vi "FPGAcode4_Test1.vi"() -> ()   [LabVIEW 2015]
uses:
  Limits_In.ctl
  Discard_Points.ctl
  Filter_Cluster.ctl
  <vilib>/Platform/TimedLoop/XDataNode/timing_clust.ctl
  <vilib>/Platform/TimedLoop/XDataNode/nitl_modes.ctl
  <vilib>/Platform/TimedLoop/XDataNode/wakeup.ctl
  Detector_Cluster.ctl
  Correlations.ctl
  <vilib>/rvi/Emulation/niFpgaGetClockAttributes.vi
  <vilib>/rvi/Emulation/niFpgaSctlEmulationGetInTimedLoop.vi
  <vilib>/rvi/Emulation/niFpgaEmulationReportErrorSimple.vi
  <vilib>/rvi/Emulation/niFpgaProcessEmulError.vi
  <vilib>/rvi/eio/common/nirviEmuTemplateMethod_errors.vi
  <vilib>/rvi/Emulation/niFpgaCriticalErrorInLSC.vi
  <vilib>/eio/EIONode/EIONode.xnode
  <vilib>/Platform/TimedLoop/XDataNode/XDataNode.xnode
  <vilib>/Platform/TimedLoop/XDataNode/XDNodeRunTimeDep.lvlib
panel:
  out "Charge":T1
  out "Mass":T2
  out "Velocity Count":T3
  in  "User Trigger Distance":fxp<+/-,34,18>
  out "User Trigger":bool
  out "Particles Discarded":i16
  out "All Discard Points":T4
  in  "Boxcar 3 Size Factor":fxp<+/-,32,16>=0.1999969482421875 format="%.2g"
  in  "Charge Error Factor":fxp<+/-,32,16>=1.100006103515625 format="%.2g"
  in  "Max Correlation Factor":fxp<+,32,4>=0.25 format="%.3g"
  in  "Threshold Factor":fxp<+/-,32,16>=1.0 format="%.2g"
  out "DCS 2":bool
  out "Detectors":cluster{"Det 1":i16, "Det 3":i16}
  out "DCS 1":bool
  in  "Limits":T6
  in  "Calibrate":bool=TRUE
  in  "Armed":bool
  out "Plates":bool
  in  "One Shot":bool
  # "These factors above are in the front\npanel so it is possible to experiment\nwith many different configurations\nof the FPGA on the fly. One can even\nchange the relative size of one filter."
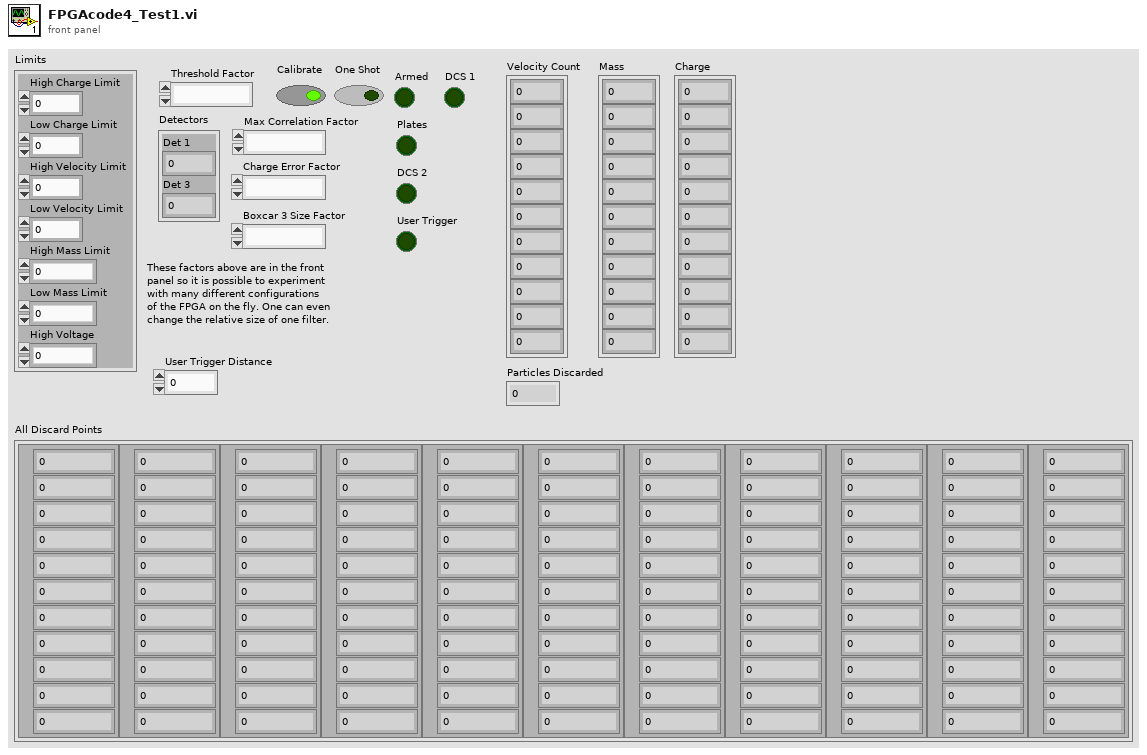
[diagram p1: front panel]
types:
  T1 = cluster{"[0]":fxp<+/-,64,-10>, "[1]":fxp<+/-,64,-10>, "[2]":fxp<+/-,64,-10>, "[3]":fxp<+/-,64,-10>, "[4]":fxp<+/-,64,-10>, "[5]":fxp<+/-,64,-10>, "[6]":fxp<+/-,64,-10>, "[7]":fxp<+/-,64,-10>, "[8]":fxp<+/-,64,-10>, "[9]":fxp<+/-,64,-10>, "[10]":fxp<+/-,64,-10>}
  T2 = cluster{"[0]":fxp<+/-,64,-2>, "[1]":fxp<+/-,64,-2>, "[2]":fxp<+/-,64,-2>, "[3]":fxp<+/-,64,-2>, "[4]":fxp<+/-,64,-2>, "[5]":fxp<+/-,64,-2>, "[6]":fxp<+/-,64,-2>, "[7]":fxp<+/-,64,-2>, "[8]":fxp<+/-,64,-2>, "[9]":fxp<+/-,64,-2>, "[10]":fxp<+/-,64,-2>}
  T3 = cluster{"[0]":i32, "[1]":i32, "[2]":i32, "[3]":i32, "[4]":i32, "[5]":i32, "[6]":i32, "[7]":i32, "[8]":i32, "[9]":i32, "[10]":i32}
  T4 = typedef "Discard_Points.ctl" = cluster{"Discard Points 1":T5, "Discard Points 2":T5, "Discard Points 3":T5, "Discard Points 4":T5, "Discard Points 5":T5, "Discard Points 6":T5, "Discard Points 7":T5, "Discard Points 8":T5, "Discard Points 9":T5, "Discard Points 10":T5, "Discard Points 11":T5}
  T5 = typedef "Filter_Cluster.ctl" = cluster{"1":i32, "2":i32, "3":i32, "4":i32, "5":i32, "6":i32, "7":i32, "8":i32, "9":i32, "10":i32, "11":i32}
  T6 = typedef "Limits_In.ctl" = cluster{"High Charge Limit":fxp<+,32,-41>, "Low Charge Limit":fxp<+,32,-41>, "High Velocity Limit":fxp<+,18,18>, "Low Velocity Limit":fxp<+,18,18>, "High Mass Limit":fxp<+/-,33,-35>, "Low Mass Limit":fxp<+/-,33,-35>, "High Voltage":fxp<+,16,22>}
  T7 = typedef "Detector_Cluster.ctl" = cluster{"Det 1":i32, "Det 2":i32}
  T8 = cluster{"Filter 1":T7, "Filter 2":T7, "Filter 3":T7, "Filter 4":T7}
  T9 = cluster{"Distance to PSU":fxp<+/-,32,5>, "Distance to end of PSU":fxp<+/-,32,5>, "Distance to DCS 2":fxp<+/-,32,5>, "Distance to DCS 1":fxp<+/-,32,5>, "Distance to front of LEIL Chamber":fxp<+/-,32,5>}
  T10 = cluster{"Detector Max Speed Count":i32, "Detector Min Speed Count":i32, "Gap Max Speed Count":i32, "Gap Min Speed Count":i32}
  T11 = cluster{"Distance to PSU":fxp<+/-,64,22>, "Distance to end of PSU":fxp<+/-,64,22>, "Distance to DCS 2":fxp<+/-,64,22>, "Distance to DCS 1":fxp<+/-,64,22>, "Distance to front of LEIL Chamber":fxp<+/-,64,22>}
  T12 = typedef "XDNodeRunTimeDep.lvlib/timing_clust.ctl" = cluster{"Expected End [f-1]":u64, "Actual End [f-1]":u64, "Finished Late? [f-1]":bool, "Expected End [i-1]":u64, "Actual End [i-1]":u64, "Finished Late? [i-1]":bool, "Expected Start [i]":u64, "Actual Start [i]":u64, "Expected Start [f]":u64, "Actual Start [f]":u64, "Source Name":string, "Structure Name":string, "Period":i64, "Deadline":i64, "Offset":i64, "Start":i64, "Priority":i32, "Timeout":i32, "Mode":T13, "Wakeup Reason":T14, "Error":errorcluster, "Source Type":string, "Secondary Source Type":string, "Global End Time":u64, "Global Start Time":u64, "Frame Duration":u64, "Iteration Duration":u64, "Assigned CPU":i32, "I/O Scan Engine Mode":u32}
  T13 = typedef "XDNodeRunTimeDep.lvlib/nitl_modes.ctl" = enum32{"No Change", "Process missed periods, maintain original phase", "Discard missed periods, maintain original phase", "Process missed periods, ignore original phase", "Discard missed periods, ignore original phase"}
  T14 = typedef "XDNodeRunTimeDep.lvlib/wakeup.ctl" = enum32{"Normal", "Aborted", "Asynchronous wakeup", "Timing source error", "Timed loop error", "Timeout"}
  T15 = cluster{"Filter 1":T7, "Filter 2":T7, "Filter 3":T7, "Filter 4":T7}[]
  T16 = cluster{"Distance to PSU":i32, "Distance to end of PSU":i32, "Distance to DCS 2":i32, "Distance to DCS 1":i32, "Distance to front of LEIL Chamber":i32}
  T17 = typedef "Correlations.ctl" = cluster{"First Correlation":i32, "Latest Correlation":i32}
  T18 = cluster{"First Detector Count":i32, "Detector Gap Count":i32, "Second Detector Count":i32, "Second Detector Final Count":i32}
  T19 = cluster{"Detectors":cluster{"Det 1":i16, "Det 3":i16}, cluster{"Det 1":i16, "Det 2":i16}, cluster{"Det 1":i16, "Det 2":i16}, cluster{"Det 1":i16, "Det 2":i16}}
  T20 = cluster{cluster{"Det 1":i16, "Det 2":i16}, cluster{"Det 1":i16, "Det 2":i16}, cluster{"Det 1":i16, "Det 2":i16}, cluster{"Det 1":i16, "Det 2":i16}}
  T21 = cluster{"[0]":u8, "[1]":u8, "[2]":u8, "[3]":u8, "[4]":u8, "[5]":u8, "[6]":u8, "[7]":u8, "[8]":u8, "[9]":u8, "[10]":u8}
  T22 = cluster{"All Discard Points[0]":T5, "All Discard Points[1]":T5, "All Discard Points[2]":T5, "All Discard Points[3]":T5, "All Discard Points[4]":T5, "All Discard Points[5]":T5, "All Discard Points[6]":T5, "All Discard Points[7]":T5, "All Discard Points[8]":T5, "All Discard Points[9]":T5, "All Discard Points[10]":T5}
  T23 = cluster{i32[], fxp<+/-,64,-2>[], fxp<+/-,64,-10>[]}
  T24 = cluster{"IO Module\\AI 0":i16, "IO Module\\AI 1":i16}
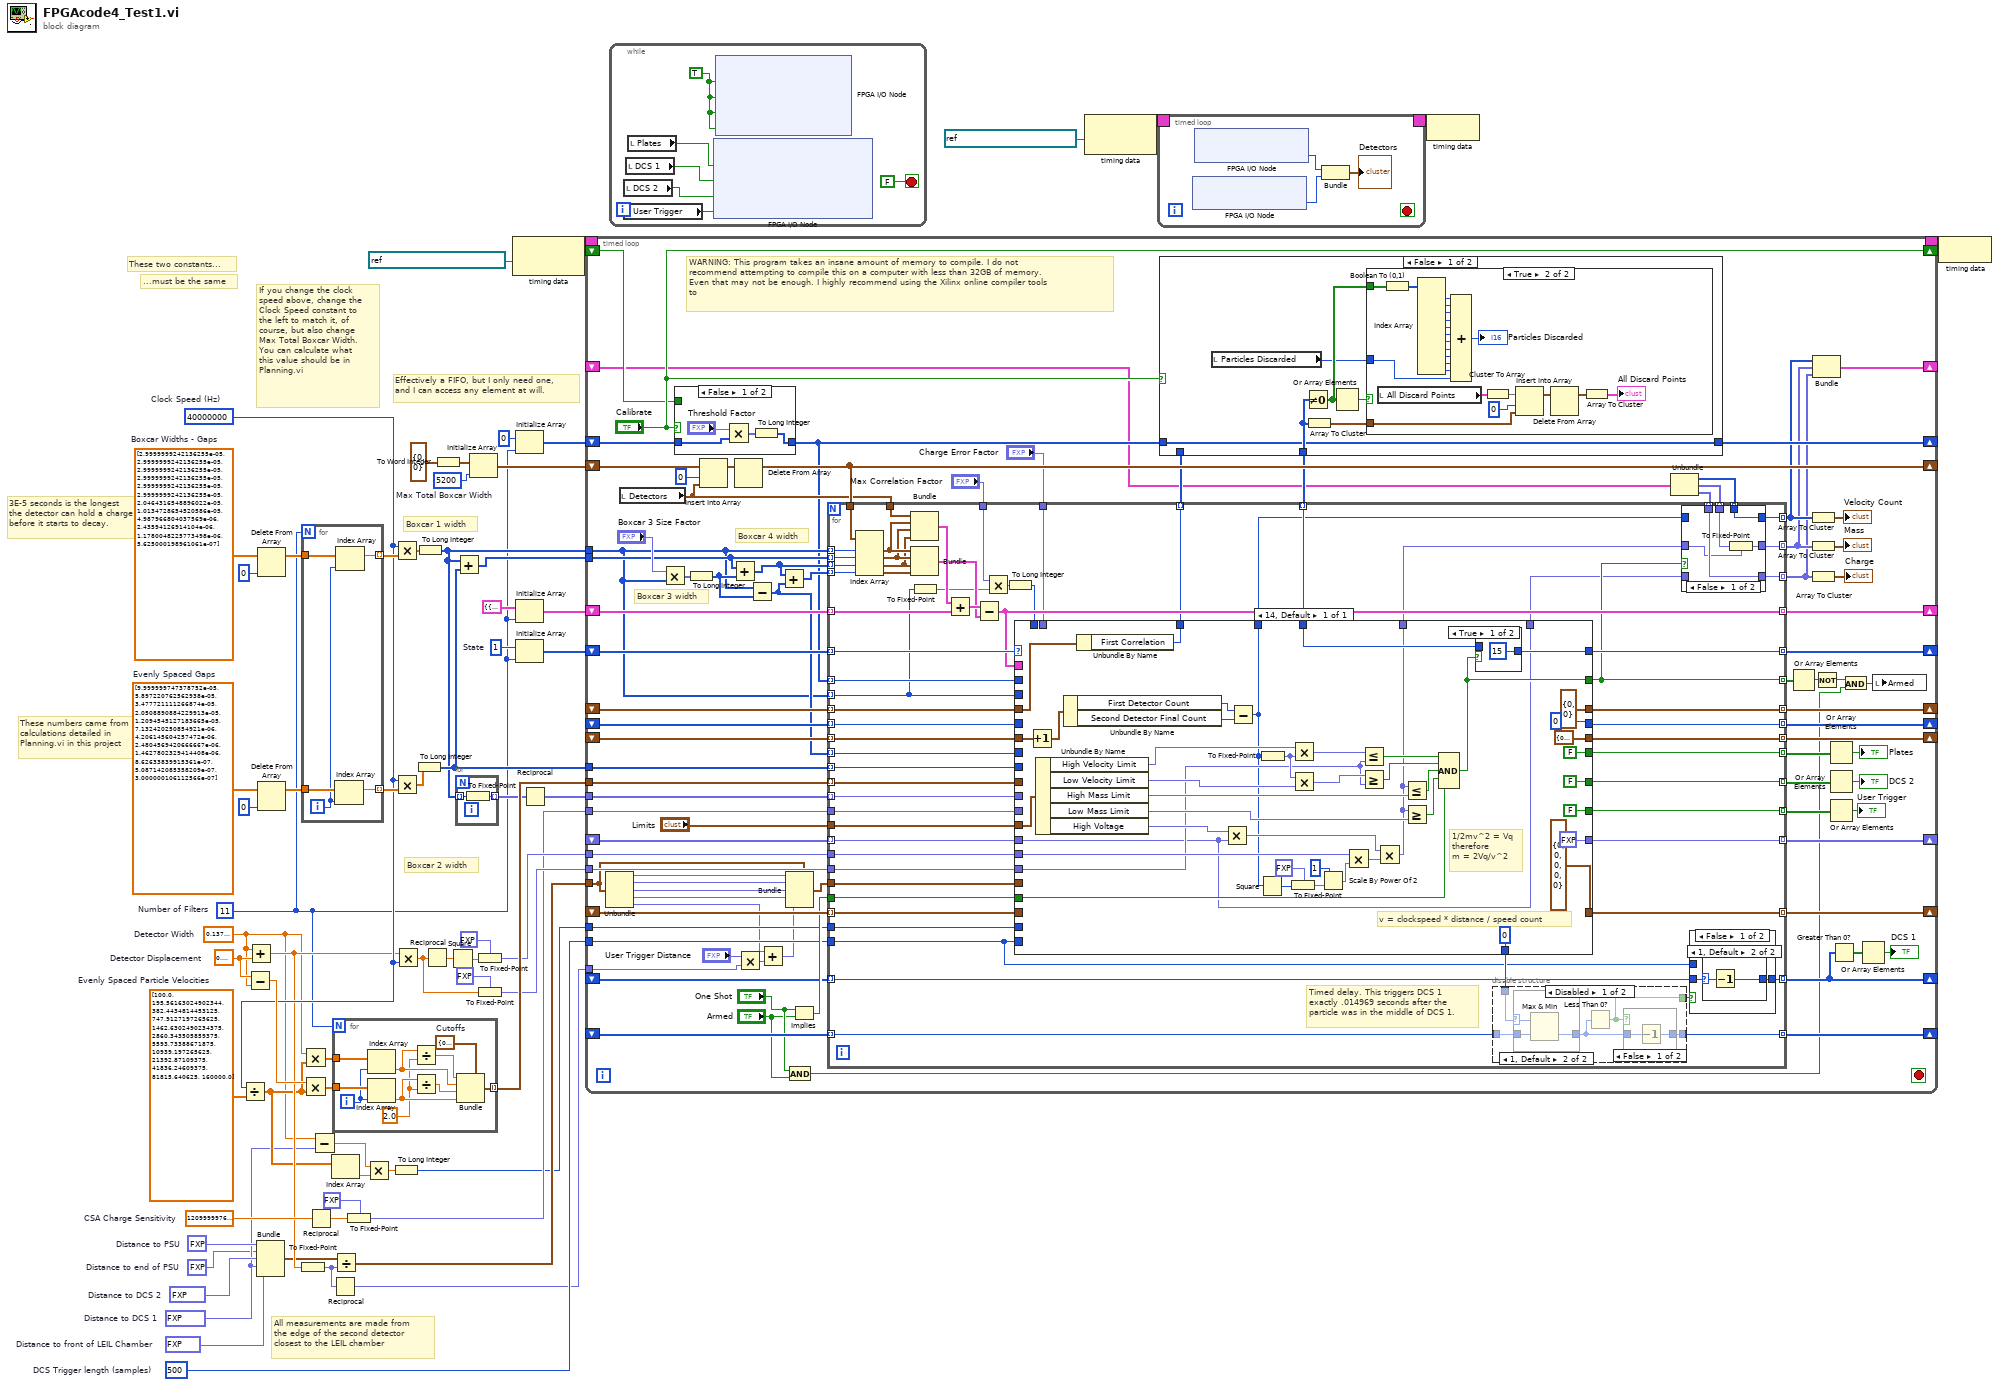
[diagram p0: block diagram]
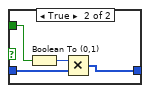
[diagram p2: hidden frame]
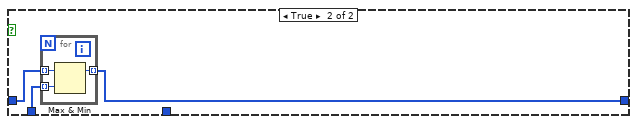
[diagram p4: hidden frame]
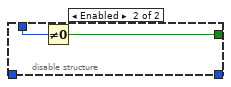
[diagram p10: hidden frame]
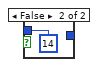
[diagram p11: hidden frame]
diagram:
  w1 = fxp<+/-,32,5> 4.297679997980595  # Distance to front of LEIL Chamber
  w7 = u16 500  # DCS Trigger length (samples)
  w12 = fxp<+/-,32,5> -1.3589000031352043  # Distance to DCS 1
  w16 = fxp<+/-,32,5> 2.6162000000476837  # Distance to DCS 2
  w4 = fxp<+/-,32,5> 1.8999999985098839  # Distance to end of PSU
  w17 = fxp<+/-,32,5> 1.5  # Distance to PSU
  w30 = sgl 12100000000000.0  # CSA Charge Sensitivity
  w52 = u8 1  # State
  w13 = sgl 0.6  # Detector Displacement
  w58 = sgl[] [3e-05, 3e-05, 3e-05, 3e-05, 3e-05, 3e-05, 2.0464317e-05, 1.0134729e-05, 4.987967e-06, 2.4359413e-06, 1.1780048e-06, 5.625e-07]  # Boxcar Widths - Gaps
  w56 = sgl[] [0.0001, 5.8972208e-05, 3.477721e-05, 2.050889e-05, 1.2094545e-05, 7.1324203e-06, 4.2061456e-06, 2.480457e-06, 1.4627802e-06, 8.6263384e-07, 5.087142e-07, 3e-07]  # Evenly Spaced Gaps
  w36 = sgl[] [100.0, 195.56163, 382.44348, 747.9127, 1462.6302, 2860.3435, 5593.734, 10939.197, 21392.871, 41836.246, 81815.64, 160000.0]  # Evenly Spaced Particle Velocities
  w33 = 40000000  # Clock Speed (Hz)
  w8 = sgl 0.138  # Detector Width
  w60 = 5200  # Max Total Boxcar Width
  w5 = 11  # Number of Filters
  # "...must be the same"
  # "These two constants..."
  # "If you change the clock\nspeed above, change the\nClock Speed constant to\nthe left to match it, of\ncourse, but also change\nMax Total Boxcar Width.\nYou can calculate what\nthis value should be in\nPlanning.vi"
  # "All measurements are made from\nthe edge of the second detector\nclosest to the LEIL chamber"
  # "Effectively a FIFO, but I only need one,\nand I can access any element at will."
  # "Boxcar 2 width"
  # "Boxcar 1 width"
  # "3E-5 seconds is the longest\nthe detector can hold a charge\nbefore it starts to decay."
  # "These numbers came from\ncalculations detailed in\nPlanning.vi in this project"
  n1 = Divide(x=w33, y=w36) -> (x/y=w14:sgl[])
  n2 = Subtract(x=w13, y=w8) -> (x-y=w35:sgl)
  n3 = Add(x=w8, y=w13) -> (x+y=w22:sgl)
  n4 = Bundle("Distance to PSU"=w17, "Distance to end of PSU"=w4, "Distance to DCS 2"=w16, "Distance to DCS 1"=w12, "Distance to front of LEIL Chamber"=w1) -> (w21:T9)  [unwired: 1 in]
  n5 = Delete From Array(array=w58, index=0) -> (array with subset deleted=w45:sgl[])  [unwired: 1 in, 1 out]
  n6 = Delete From Array(array=w56, index=0) -> (array with subset deleted=w47:sgl[])  [unwired: 1 in, 1 out]
  n7 = To Fixed-Point(number=w22) -> (fixed-point=w3:fxp<+/-,32,16>)  [unwired: 1 in]
  n8 = for {
    N: w5 -> [_]
    tunnel: w47 -> [w72]
    tunnel: [w69] -> w46 mode=indexing
    tunnel: w45 -> [w71]
    tunnel: [w70] -> w44 mode=indexing
    i -> [w68]
    n9 = Index Array(array=w72, index=w68) -> (element=w69:sgl)
    n10 = Index Array(array=w71, index=w68) -> (element=w70:sgl)
  }
  n11 = Multiply(x=w8, y=w14) -> (x*y=w54:sgl[])
  n12 = Multiply(x=w35, y=w14) -> (x*y=w55:sgl[])
  n13 = Reciprocal(x=w30) -> (1/x=w24:sgl)
  n14 = Subtract(x=w8, y=w12) -> (x-y=w10:sgl)
  n15 = Index Array(array=w14) -> (element=w11:sgl)  [unwired: 1 in]
  n16 = Reciprocal(x=w3) -> (1/x=w2:fxp<+/-,34,18>)
  n17 = for {
    N: w5 -> [_]
    tunnel: w55 -> [w82]
    tunnel: w54 -> [w81]
    tunnel: [w80] -> w49 mode=indexing
    i -> [w79]
    w73 = sgl 2.0 ("y")
    w78 = T10 {"Detector Max Speed Count"=0, "Detector Min Speed Count"=0, "Gap Max Speed Count"=0, "Gap Min Speed Count"=0}  # Cutoffs
    n18 = Index Array(array=w81, index=w79) -> (element=w77:sgl)
    n19 = Index Array(array=w82, index=w79) -> (element=w74:sgl)
    n20 = Divide(x=w77, y=w73) -> (x/y=w76:sgl)
    n21 = Divide(x=w74, y=w73) -> (x/y=w75:sgl)
    n22 = Bundle(cluster=w78, "Detector Max Speed Count"=w76, "Detector Min Speed Count"=w77, "Gap Max Speed Count"=w75, "Gap Min Speed Count"=w74) -> (w80:T10)
  }
  n23 = Divide(x=w21, y=w3) -> (x/y=w20:T11)
  n24 = To Fixed-Point(fixed-point type=fxp<+,32,-43> 0.0, number=w24) -> (fixed-point=w23:fxp<+,32,-43>)
  n25 = Multiply(x=w10, y=w11) -> (x*y=w9:sgl)
  n26 = To Long Integer(number=w9) -> (32bit integer=w6:i32)
  n27 = Multiply(x=w33, y=w44) -> (x*y=w48:sgl[])
  n28 = Multiply(x=w33, y=w46) -> (x*y=w53:sgl[])
  n29 = Multiply(x=w22, y=w33) -> (x*y=w27:sgl)
  n30 = To Long Integer(number=w53) -> (32bit integer=w43:i32[])
  n31 = To Long Integer(number=w48) -> (32bit integer=w39:i32[])
  n32 = Reciprocal(x=w27) -> (1/x=w32:sgl)
  n33 = To Word Integer(number=T7 {"Det 1"=0, "Det 2"=0} ("Detectors")) -> (16bit integer=w42:cluster{"Det 1":i16, "Det 2":i16})
  n34 = Square(x=w32) -> (x^2=w31:sgl)
  n35 = Add(x=w39, y=w43) -> (x+y=w15:i32[])
  n36 = for {
    tunnel: w39 -> [w84] mode=indexing
    tunnel: [w83] -> w38 mode=indexing
    n37 = To Fixed-Point(number=w84) -> (fixed-point=w83:fxp<+/-,32,32>)  [unwired: 1 in]
  }
  n38 = Initialize Array(w42, w60) -> (w61:cluster{"Det 1":i16, "Det 2":i16}[])
  n39 = To Fixed-Point(fixed-point type=fxp<+/-,32,-45> 0.0, number=w31) -> (fixed-point=w34:fxp<+/-,32,-45>)
  n40 = To Fixed-Point(fixed-point type=fxp<+,32,32> 0.0, number=w27) -> (fixed-point=w25:fxp<+,32,32>)
  n41 = node-c288(refnum<k21> "40 MHz Onboard Clock" ("Source Name")) -> (w64:T12)
  n42 = Initialize Array(0 ("element"), w5) -> (w18:i32[])
  n43 = Initialize Array(T8 {"Filter 1"={"Det 1"=0, "Det 2"=0}, "Filter 2"={"Det 1"=0, "Det 2"=0}, "Filter 3"={"Det 1"=0, "Det 2"=0}, "Filter 4"={"Det 1"=0, "Det 2"=0}} ("cluster"), w5) -> (w50:T15)
  n44 = Initialize Array(w52, w5) -> (w51:u8[])
  n45 = Reciprocal(x=w38) -> (1/x=w37:fxp<+/-,34,2>[])
  n46 = timed-loop {
    timing: w64 -> [_]
    timing-out: [_] -> w63
    shift-right: [w168] -> _
    shift-left: w61 -> [w171]
    shift-right: [w167] -> _
    shift-left: w50 -> [w160]
    shift-right: [w165] -> _
    shift-left: w51 -> [w166]
    shift-right: [w164] -> _
    shift-left: _ -> [w163]
    shift-right: [w162] -> _
    shift-left: _ -> [w161]
    tunnel: w49 -> [w158]
    shift-right: [w157] -> _
    shift-left: _ -> [w156]
    tunnel: w39 -> [w145]
    tunnel: w15 -> [w151]
    tunnel: w43 -> [w146]
    tunnel: w37 -> [w144]
    shift-right: [w142] -> _
    shift-left: _ -> [w141]
    tunnel: w34 -> [w140]
    tunnel: w23 -> [w139]
    tunnel: w25 -> [w138]
    tunnel: w20 -> [w116]
    shift-right: [w137] -> _
    shift-left: _ -> [w136]
    shift-right: [w134] -> _
    shift-left: w18 -> [w132]
    shift-right: ["Calibrate"] -> _
    shift-left: _ -> [w129]
    tunnel: w7 -> [w127]
    tunnel: w6 -> [w126]
    shift-right: [w123] -> _
    shift-left: _ -> [w125]
    shift-right: [w121] -> _
    shift-left: _ -> [w120]
    tunnel: w2 -> [w119]
    shift-right: [w90] -> _
    shift-left: _ -> [w89]
    stop <- _ stop-if-true
    # "WARNING: This program takes an insane amount of memory to compile. I do not\nrecommend attempting to compile this on a computer with less than 32GB of memory.\nEven that may not be enough. I highly recommend using the Xilinx online compiler tools\nto"
    # "Boxcar 3 width"
    # "Boxcar 4 width"
    n47 = Unbundle(w116) -> ("Distance to PSU"=w117:fxp<+/-,64,22>, "Distance to end of PSU"=w115:fxp<+/-,64,22>, "Distance to DCS 2"=w114:fxp<+/-,64,22>, "Distance to DCS 1"=w111:fxp<+/-,64,22>, "Distance to front of LEIL Chamber"=w110:fxp<+/-,64,22>)
    n48 = local read "Detectors"() -> (w159:cluster{"Det 1":i16, "Det 3":i16})
    n49 = Multiply(x="Boxcar 3 Size Factor", y=w145) -> (x*y=w153:fxp<+/-,64,48>[])
    n50 = case shown="False" "Calibrate" {
      tunnel: w132 -> [w173 w179]
      tunnel: [w172 w177] -> w131
      tunnel: w129 -> [_ w178]
      frame False {
        n51 = Multiply(x="Threshold Factor", y=w173) -> (x*y=w174:fxp<+/-,64,48>[])
        n52 = To Long Integer(number=w174) -> (32bit integer=w172:i32[])
      }
      frame True {
        n53 = Boolean To (0,1)(Boolean=w178) -> (0, 1=w176:i16)
        n54 = Multiply(x=w176, y=w179) -> (x*y=w177:i32[])
      }
    }
    n55 = To Long Integer(number=w153) -> (32bit integer=w154:i32[])
    n56 = Insert Into Array(array=w171, index=0, new element=w159) -> (w170:cluster{"Det 1":i16, "Det 2":i16}[])
    n57 = Add(x=w151, y=w154) -> (x+y=w150:i32[])
    n58 = Delete From Array(array=w170) -> (array with subset deleted=w168:cluster{"Det 1":i16, "Det 2":i16}[])  [unwired: 2 in, 1 out]
    n59 = Multiply(x="User Trigger Distance", y=w119) -> (x*y=w112:fxp<+/-,64,34>)
    n60 = Subtract(x=w145, y=w154) -> (x-y=w148:i32[])
    n61 = Add(x=w110, y=w112) -> (x+y=w109:fxp<+/-,64,35>)
    n62 = Add(x=w150, y=w148) -> (x+y=w149:i32[])
    n63 = Bundle(cluster=w116, "Distance to PSU"=w117, "Distance to end of PSU"=w115, "Distance to DCS 2"=w114, "Distance to DCS 1"=w111, "Distance to front of LEIL Chamber"=w109) -> (w113:T11)
    n64 = And(x="One Shot", y="Armed") -> (x .and. y?=w99:bool)
    n65 = Implies(1:"Armed", 2:"One Shot") -> (0:w128:bool)
    n66 = Unbundle(w89) -> (w88:i32[], w87:fxp<+/-,64,-2>[], w86:fxp<+/-,64,-10>[])
    n67 = for {
      tunnel: w168 -> [w280]
      tunnel: [w263] -> w167 mode=indexing
      tunnel: w166 -> [w279] mode=indexing
      tunnel: [w277] -> w165 mode=indexing
      tunnel: w131 -> [w278] mode=indexing
      tunnel: [w276] -> w164 mode=indexing
      tunnel: w163 -> [w275] mode=indexing
      tunnel: [w274] -> w162 mode=indexing
      tunnel: w161 -> [w273] mode=indexing
      tunnel: w160 -> [w267] mode=indexing
      tunnel: w159 -> [w272]
      tunnel: w158 -> [w262] mode=indexing
      tunnel: [w261] -> w157 mode=indexing
      tunnel: w156 -> [w260] mode=indexing
      tunnel: w145 -> [w259] mode=indexing
      tunnel: w151 -> [w258] mode=indexing
      tunnel: w150 -> [w257] mode=indexing
      tunnel: w149 -> [w256] mode=indexing
      tunnel: w145 -> [w216] mode=indexing
      tunnel: "Max Correlation Factor" -> [w255]
      tunnel: w148 -> [w254] mode=indexing
      tunnel: w146 -> [w253] mode=indexing
      tunnel: "Charge Error Factor" -> [w252]
      tunnel: [w251] -> w135 mode=indexing
      tunnel: w144 -> [w250] mode=indexing
      tunnel: "Limits" -> [w249]
      tunnel: [w248] -> w142 mode=indexing
      tunnel: w141 -> [w247] mode=indexing
      tunnel: w140 -> [w246]
      tunnel: w139 -> [w245]
      tunnel: w138 -> [w244]
      tunnel: w113 -> [w243]
      tunnel: [w242] -> w137 mode=indexing
      tunnel: w136 -> [w241] mode=indexing
      tunnel: [w240] -> w133 mode=indexing
      tunnel: w128 -> [w239]
      tunnel: w127 -> [w236]
      tunnel: w126 -> [w238]
      tunnel: [w235] -> w123 mode=indexing
      tunnel: w125 -> [w234] mode=indexing
      tunnel: [w232] -> w121 mode=indexing
      tunnel: w120 -> [w231] mode=indexing
      tunnel: [w230] -> w108 mode=indexing
      tunnel: [w229] -> w106 mode=indexing
      tunnel: [w228] -> w105 mode=indexing
      tunnel: [w227] -> w102 mode=indexing
      tunnel: [w221] -> w93 mode=indexing
      tunnel: [w226] -> w91 mode=indexing
      tunnel: [w224] -> w92 mode=indexing
      tunnel: w88 -> [w220] mode=indexing
      tunnel: w87 -> [w219] mode=indexing
      tunnel: w86 -> [w218] mode=indexing
      # "Timed delay. This triggers DCS 1\nexactly .014969 seconds after the\nparticle was in the middle of DCS 1."
      n68 = Index Array(array=w280, index #1=w259, index #2=w258, index #3=w257, index #4=w256) -> (element #1=w270:cluster{"Det 1":i16, "Det 2":i16}, element #2=w269:cluster{"Det 1":i16, "Det 2":i16}, element #3=w268:cluster{"Det 1":i16, "Det 2":i16}, element #4=w271:cluster{"Det 1":i16, "Det 2":i16})
      n69 = Bundle("Detectors"=w272, w270, w269, w268) -> (w266:T19)  [unwired: 1 in]
      n70 = Bundle(w270, w269, w268, w271) -> (w264:T20)  [unwired: 1 in]
      n71 = To Fixed-Point(number=w216) -> (fixed-point=w215:fxp<+/-,32,32>)  [unwired: 1 in]
      n72 = Add(x=w266, y=w267) -> (x+y=w265:T8)
      n73 = Subtract(x=w265, y=w264) -> (x-y=w263:T8)
      n74 = Multiply(x=w255, y=w215) -> (x*y=w217:fxp<+/-,64,36>)
      n75 = To Long Integer(number=w217) -> (32bit integer=w214:i32)
      n76 = case shown="14, Default" w279 {
        tunnel: w278 -> [_]
        tunnel: [w331] -> w277
        tunnel: w216 -> [_]
        tunnel: [T17 {"First Correlation"=0, "Latest Correlation"=0} ("input cluster")] -> w276
        tunnel: w275 -> [w323]
        tunnel: [0] -> w274
        tunnel: w273 -> [_]
        tunnel: w263 -> [_]
        tunnel: w262 -> [_]
        tunnel: [T18 {"First Detector Count"=0, "Detector Gap Count"=0, "Second Detector Count"=0, "Second Detector Final Count"=0} ("Cutoffs")] -> w261
        tunnel: w260 -> [w350]
        tunnel: w214 -> [_]
        tunnel: w254 -> [_]
        tunnel: w253 -> [_]
        tunnel: w252 -> [_]
        tunnel: [w330] -> w251
        tunnel: w250 -> [_]
        tunnel: w249 -> [w351]
        tunnel: [fxp<+/-,64,-10> 0.0] -> w248
        tunnel: w247 -> [w318]
        tunnel: w246 -> [w344]
        tunnel: w245 -> [_]
        tunnel: w244 -> [w324]
        tunnel: w243 -> [_]
        tunnel: [T16 {"Distance to PSU"=0, "Distance to end of PSU"=0, "Distance to DCS 2"=0, "Distance to DCS 1"=0, "Distance to front of LEIL Chamber"=0}] -> w242
        tunnel: w241 -> [_]
        tunnel: [w322] -> w240
        tunnel: w239 -> [w321]
        tunnel: w238 -> [_]
        tunnel: w236 -> [_]
        tunnel: [0] -> w237
        tunnel: [FALSE] -> w230
        tunnel: [FALSE] -> w229
        tunnel: [FALSE] -> w228
        tunnel: [w320] -> w227
        tunnel: [w319] -> w222
        tunnel: [w318] -> w225
        tunnel: [w317] -> w223
        frame 14, Default {
          # "v = clockspeed * distance / speed count"
          # "1/2mv^2 = Vq\ntherefore\nm = 2Vq/v^2"
          n77 = Increment(x=w350) -> (x+1=w349:T18)
          n78 = Unbundle By Name(w351) -> ("High Velocity Limit"=w328:fxp<+,18,18>, "Low Velocity Limit"=w329:fxp<+,18,18>, "High Mass Limit"=w339:fxp<+/-,33,-35>, "Low Mass Limit"=w340:fxp<+/-,33,-35>, "High Voltage"=w334:fxp<+,16,22>)
          n79 = Unbundle By Name(w349) -> ("First Detector Count"=w348:i32, "Second Detector Final Count"=w347:i32)
          n80 = Unbundle By Name(w323) -> ("First Correlation"=w322:i32)
          n81 = Multiply(x=w334, y=w318) -> (x*y=w341:fxp<+/-,64,12>)
          n82 = Subtract(x=w348, y=w347) -> (x-y=w319:i32)
          n83 = Square(x=w319) -> (x^2=w346:i32)
          n84 = To Fixed-Point(number=w319) -> (fixed-point=w327:fxp<+/-,32,32>)  [unwired: 1 in]
          n85 = To Fixed-Point(fixed-point type=fxp<+,32,32> 0.0, number=w346) -> (fixed-point=w343:fxp<+,32,32>)
          n86 = Multiply(x=w328, y=w327) -> (x*y=w326:fxp<+/-,50,50>)
          n87 = Multiply(x=w327, y=w329) -> (x*y=w325:fxp<+/-,50,50>)
          n88 = Scale By Power Of 2(n=i16 1, x=w343) -> (x*2^n=w333:fxp<+,32,32>)
          n89 = Multiply(x=w344, y=w333) -> (x*y=w342:fxp<+/-,64,-13>)
          n90 = Less Or Equal?(x=w326, y=w324) -> (x <= y?=w338:bool)
          n91 = Greater Or Equal?(x=w325, y=w324) -> (x >= y?=w337:bool)
          n92 = Multiply(x=w341, y=w342) -> (x*y=w317:fxp<+/-,64,-2>)
          n93 = Less Or Equal?(x=w317, y=w339) -> (x <= y?=w336:bool)
          n94 = Greater Or Equal?(x=w317, y=w340) -> (x >= y?=w335:bool)
          n95 = Compound Arithmetic op=AND(w338, w337, w336, w335, w321) -> (w320:bool)
          n96 = case shown="True" w320 {
            tunnel: [u8 15 ("Det 3") _] -> w331
            tunnel: [_ u8 14 ("Det 3")] -> w330
            frame True {
            }
            frame False {
            }
          }
        }
      }
      n97 = disable-structure shown="Disabled" {
        disable-tunnel: w237 -> [w299 w307]
        disable-tunnel: [w295 w306] -> w233
        disable-tunnel: [w297 _] -> w232
        disable-tunnel: w231 -> [w298 _]
        frame Disabled {
          n98 = case shown="1, Default" w299 {
            selector: w299 -> [_ w305]
            tunnel: [w302 w303] -> w296
            tunnel: w298 -> [w302 w304]
            frame 0 {
            }
            frame 1, Default {
              n99 = Max & Min(x=w305, y=w304) -> (min(x,y)=w303:i32)  [unwired: 1 out]
            }
          }
          n100 = Less Than 0?(x=w296) -> (x < 0?=w295:bool)
          n101 = case shown="False" w295 {
            tunnel: w296 -> [w301 _]
            tunnel: [w300 _] -> w297
            frame False {
              n102 = Decrement(x=w301) -> (x-1=w300:i32)
            }
            frame True {
            }
          }
        }
        frame Enabled {
          n103 = Not Equal To 0?(x=w307) -> (x != 0?=w306:bool)
        }
      }
      n104 = case shown="False" w227 {
        tunnel: [w284 w288] -> w226
        tunnel: w225 -> [_ w288]
        tunnel: [w282 w286] -> w224
        tunnel: w223 -> [w281 w286]
        tunnel: w222 -> [_ w287]
        tunnel: [w285 w287] -> w221
        tunnel: w220 -> [w285 _]
        tunnel: w219 -> [w283 _]
        tunnel: w218 -> [w284 _]
        frame False {
          n105 = To Fixed-Point(fixed-point type=w281, number=w283) -> (fixed-point=w282:fxp<+/-,64,-2>)
        }
        frame True {
        }
      }
      n106 = case shown="False" w233 {
        tunnel: w236 -> [_ w294]
        tunnel: [w289 w294] -> w235
        tunnel: w234 -> [w290 _]
        frame False {
          n107 = case shown="1, Default" w290 {
            selector: w290 -> [w291 w293]
            tunnel: [w291 w292] -> w289
            frame 0 {
            }
            frame 1, Default {
              n108 = Decrement(x=w293) -> (x-1=w292:u16)
            }
          }
        }
        frame True {
        }
      }
    }
    n109 = case shown="False" "Calibrate" {
      tunnel: w135 -> [w184 _]
      tunnel: w131 -> [w180 w210]
      tunnel: [w180 w208] -> w134
      tunnel: w133 -> [_ w209]
      frame False {
        n110 = local read "Particles Discarded"() -> (w182:i16)
        n111 = Not Equal To 0?(x=w184) -> (x != 0?=w183:bool[])
        n112 = Array To Cluster(array=w184) -> (cluster=w185:T21)
        n113 = Or Array Elements(Boolean array=w183) -> (logical OR=w181:bool)
        n114 = case shown="True" w181 {
          tunnel: w185 -> [_ w201]
          tunnel: w183 -> [_ w187]
          tunnel: w182 -> [_ w186]
          frame False {
          }
          frame True {
            n115 = local read "All Discard Points"() -> (w207:T4)
            n116 = Boolean To (0,1)(Boolean=w187) -> (0, 1=w188:i16[])
            n117 = Index Array(array=w188) -> (element #1=w190:i16, element #2=w191:i16, element #3=w192:i16, element #4=w193:i16, element #5=w194:i16, element #6=w195:i16, element #7=w196:i16, element #8=w197:i16, element #9=w198:i16, element #10=w199:i16, element #11=w189:i16)  [unwired: 11 in]
            n118 = Compound Arithmetic op=ADD(w190, w191, w192, w193, w194, w195, w196, w197, w198, w199, w189, w186) -> (→"Particles Discarded":i16)
            n119 = Cluster To Array(cluster=w207) -> (array=w203:T5[])
            n120 = Insert Into Array(array=w203, index=0, new element=w201) -> (w205:T5[])
            n121 = Delete From Array(array=w205) -> (array with subset deleted=w202:T5[])  [unwired: 2 in, 1 out]
            n122 = Array To Cluster(array=w202) -> (cluster=→"All Discard Points":T22)
          }
        }
      }
      frame True {
        n123 = for {
          tunnel: w209 -> [w213] mode=indexing
          tunnel: w210 -> [w212] mode=indexing
          tunnel: [w211] -> w208 mode=indexing
          n124 = Max & Min(x=w212, y=w213) -> (max(x,y)=w211:i32)  [unwired: 1 out]
        }
      }
    }
    n125 = Or Array Elements(Boolean array=w102) -> (logical OR=w96:bool)
    n126 = Array To Cluster(array=w93) -> (cluster=→"Velocity Count":T3)
    n127 = Array To Cluster(array=w92) -> (cluster=→"Mass":T2)
    n128 = Array To Cluster(array=w91) -> (cluster=→"Charge":T1)
    n129 = Bundle(w93, w92, w91) -> (w90:T23)  [unwired: 1 in]
    n130 = Not(x=w96) -> (.not. x?=w101:bool)
    n131 = Or Array Elements(Boolean array=w108) -> (logical OR=→"Plates":bool)
    n132 = Or Array Elements(Boolean array=w106) -> (logical OR=→"DCS 2":bool)
    n133 = Or Array Elements(Boolean array=w105) -> (logical OR=→"User Trigger":bool)
    n134 = Greater Than 0?(x=w123) -> (x > 0?=w122:bool[])
    n135 = And(x=w101, y=w99) -> (x .and. y?=w100:bool)
    n136 = Or Array Elements(Boolean array=w122) -> (logical OR=→"DCS 1":bool)
    n137 = local write "Armed"(w100) -> ()
  }
  n138 = while {
    stop <- FALSE stop-if-true
    w357 = TRUE ("IO Module\\PFI Enable")
    n139 = local read "DCS 2"() -> (w358:bool)
    n140 = local read "User Trigger"() -> (w356:bool)
    n141 = local read "DCS 1"() -> (w359:bool)
    n142 = local read "Plates"() -> (w360:bool)
    n143 = xnode "FPGA I/O Node"("IO Module\\PFI 0 Wr Data"=w360, "IO Module\\PFI 1 Wr Data"=w359, "IO Module\\PFI 2 Wr Data"=w358, "IO Module\\PFI 3 Wr Data"=w356) -> ()  [unwired: 4 in, 4 out]
    n144 = xnode "FPGA I/O Node"("IO Module\\PFI 0 WE"=w357, "IO Module\\PFI 1 WE"=w357, "IO Module\\PFI 2 WE"=w357, "IO Module\\PFI 3 WE"=w357) -> ()  [unwired: 4 in, 4 out]
  }
  n145 = node-c288(refnum<k21> "IO Module\\Data Clock" ("Source Name")) -> (w67:T12)
  n146 = timed-loop {
    timing: w67 -> [_]
    timing-out: [_] -> w66
    stop <- _ stop-if-true
    n147 = xnode "FPGA I/O Node"() -> ("IO Module\\AI 1"=w363:i16)  [unwired: 1 in, 1 out]
    n148 = xnode "FPGA I/O Node"() -> ("IO Module\\AI 0"=w364:i16)  [unwired: 1 in, 1 out]
    n149 = Bundle("IO Module\\AI 0"=w364, "IO Module\\AI 1"=w363) -> (→"Detectors":T24)  [unwired: 1 in]
  }
  n150 = node-c288(w66) -> ()
  n151 = node-c288(w63) -> ()
